vi "Verify error.vi"(8 "error in (no error)":errorcluster, 11 "Channel in":refnum<class "Channel.lvclass">) -> (0 "error out":errorcluster, 2 "error":bool, 3 "Channel out":refnum<class "Channel.lvclass">)   [LabVIEW 2018, in "Channel.lvclass"]
doc: "Verify if there is an error in the error array of the camera class\n\nThis function will return true if there is any error or warning in the error array of the camera with a code different of 20002 or 0."
uses:
  Channel.lvclass
  Channel.lvclass/Channel.ctl
  Simulated_CCD_Camera/Simulated_CCD_Camera.lvclass/Simulated_CCD_Camera.ctl
  Simulated_CCD_Camera/Simulated_CCD_Camera.lvclass
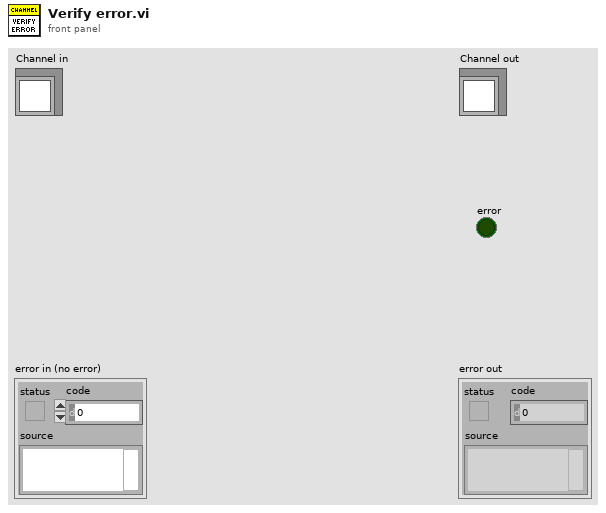
[diagram p1: front panel]
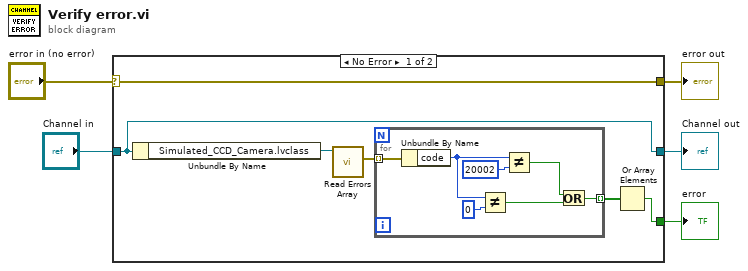
[diagram p0: block diagram]
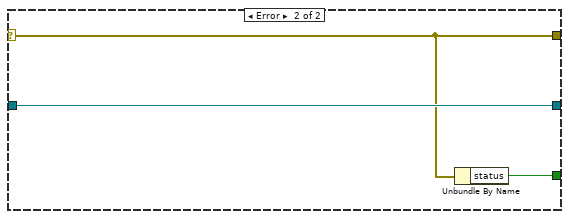
[diagram p2: hidden frame]
diagram:
  n1 = case shown="No Error" "error in (no error)" {
    selector: "error in (no error)" -> [w8 w20]
    tunnel: [w8 w20] -> w4
    tunnel: [w11 w21] -> w2
    tunnel: "Channel in" -> [w11 w21]
    tunnel: [w6 w19] -> w1
    frame No Error {
      n2 = Unbundle By Name(w11) -> ("Simulated_CCD_Camera.lvclass"=w10:refnum<class "Simulated_CCD_Camera.lvclass">)
      n3 = call "Read Errors Array.vi"("Simulated_CCD_Camera in"=w10) -> ("Errors array"=w9:errorcluster[])  [unwired: 8 in, 2 out]
      n4 = for {
        tunnel: w9 -> [w18] mode=indexing
        tunnel: [w12] -> w7 mode=indexing
        n5 = Unbundle By Name(w18) -> ("code"=w16:i32)
        n6 = Not Equal?(x=w16, y=0) -> (x != y?=w14:bool)
        n7 = Not Equal?(x=w16, y=20002) -> (x != y?=w13:bool)
        n8 = Or(x=w13, y=w14) -> (x .or. y?=w12:bool)
      }
      n9 = Or Array Elements(Boolean array=w7) -> (logical OR=w6:bool)
    }
    frame Error {
      n10 = Unbundle By Name(w20) -> ("status"=w19:bool)
    }
  }
  "error out" <- w4
  "Channel out" <- w2
  "error" <- w1
